vi "Reactor.vi"() -> ()   [LabVIEW 2017]
uses:
  <vilib>/Platform/TimedLoop/XDataNode/timing_clust.ctl
  <vilib>/Platform/TimedLoop/XDataNode/nitl_modes.ctl
  <vilib>/Platform/TimedLoop/XDataNode/wakeup.ctl
  <vilib>/Analysis/baseanly.llb/Mean (DBL).vi
  <vilib>/Utility/file.llb/Read Delimited Spreadsheet (DBL).vi
  <vilib>/platform/TimedLoop/XDataNode/XDataNode.xnode
  <vilib>/Analysis/NI_AALBase.lvlib
  <vilib>/Platform/TimedLoop/XDataNode/XDNodeRunTimeDep.lvlib
panel:
  in  "stop":bool
  in  "Controller":string(combo)
  in  "Controller\nReset":bool
  out "Server Connection":bool
  in  "Stop Reading":bool
  out "System Time [s]":sgl
  out "Power Output":dbl(graph)
  out "Frequency [Hz]":sgl(slide) scale=0.0..60.0
  out "Frequency [Hz]":sgl(slide) scale=0.0..60.0
  out "Frequency [Hz]":sgl(knob) scale=0.0..45.0
  out "Power [W]":dbl(slide) caption="Power Output [W]" scale=0.0..10000.0
  in  "Desired Power [W]":dbl format="%.1f"
  out "WT-10":sgl format="%.1f"
  out "BT-11":sgl format="%.1f"
  out "BT-12":sgl format="%.1f"
  out "WT-13":sgl format="%.1f"
  out "CX-10":dbl format="%.1f"
  out "CX-11":dbl format="%.1f"
  out "WT-20":sgl format="%.1f"
  out "BT-21":sgl format="%.1f"
  out "WT-22":sgl format="%.1f"
  out "BT-23":sgl format="%.1f"
  out "WT-24":sgl format="%.1f"
  out "BT-25":sgl format="%.1f"
  out "WT-26":sgl format="%.1f"
  out "BT-27":sgl format="%.1f"
  out "WT-28":sgl format="%.1f"
  out "BT-29":sgl format="%.1f"
  out "BT-30":sgl format="%.1f"
  out "WT-31":sgl format="%.1f"
  out "BT-32":sgl format="%.1f"
  out "WT-33":sgl format="%.1f"
  out "BT-34":sgl format="%.1f"
  out "WT-35":sgl format="%.1f"
  out "WT-40":sgl format="%.1f"
  out "BT-41":sgl format="%.1f"
  out "WT-42":sgl format="%.1f"
  out "BT-43":sgl format="%.1f"
  out "BT-60":sgl format="%.1f"
  out "WT-61":sgl format="%.1f"
  out "WT-62":sgl format="%.1f"
  out "BT-63":sgl format="%.1f"
  out "WT-64":sgl format="%.1f"
  out "BT-65":sgl format="%.1f"
  out "BT-66":sgl format="%.1f"
  out "WT-67":sgl format="%.1f"
  out "ST-10":sgl format="%.1f"
  out "ST-11":sgl format="%.1f"
  out "ST-12":sgl[](array[numeric]) format="%.1f"
  out "ST-13":sgl format="%.1f"
  out "ST-14":sgl[](array[numeric]) format="%.1f"
  out "AT-01":sgl format="%.1f"
  out "AT-02":sgl format="%.1f"
  in  "Power Output On":bool
  in  "ACTIVATE - CTAH":bool
  in  "CTAH Frequency [Hz]":sgl format="%.1f"
  in  "ACTIVATE - TCHX":bool
  in  "TCHX Frequency [Hz]":sgl format="%.1f"
  in  "ACTIVATE - PUMP":bool
  in  "Pump Frequency [Hz]":sgl format="%.1f"
  out "DHX Primary Flow\n\n\nFM-20 [kg/s]":sgl format="%.3f"
  out "Bypass Flow\n\n\nFM-30 [kg/s]":sgl format="%.3f"
  out "Primary Flow\n\n\nFM-40 [kg/s]":sgl format="%.3f"
  out "DRACS Flow\n\n\nFM-60 [kg/s]":sgl format="%.3f"
  in  "Flow Data?":bool=TRUE
  out "System Safe":bool
  in  "Exit Profile":bool
  in  "Select Operation Mode":T1(ring) caption="Select Operation Mode2"
  out "System Loop Time (ms)":u32
  in  "Load Power Profile":bool
  in  "Dyn. Power Profile File":path
  out "CTAH Temperatures":cluster{"CTAH Outlet":dbl, "CTAH Inlet":dbl}(graph)
  out "CTAH Outlet":dbl format="%0.2f"
  out "CTAH Inlet":dbl format="%0.2f"
  out "Core Temperatures":cluster{"Heater Inlet":dbl, "Heater Outlet":dbl}(graph)
  out "Heater Outlet":dbl format="%0.2f"
  out "Heater Inlet":dbl format="%0.2f"
  out "Profile Step":i32
  out "Power Input Signal [W]":dbl
  out "Output Current 2 [A]":dbl
  out "Output Voltage 2 [V]":dbl
  out "Output Current 1 [A]":dbl
  out "Output Voltage 1 [V]":dbl
  out "Loop Period [ms]":i64
  in  "Pump Operation Mode":i32(listbox)
  in  "TCHX Operation Mode":i32(listbox)
  in  "CTAH Operation Mode":i32(listbox)
  in  "Stop Reactor Interface":bool
  # "DRACS"
  # "PRIMARY"
  # "HOT DRACS"
  # "TCHX"
  # "HOT LEG"
  # "DHX TOP"
  # "N"
  # "COLD DRACS"
  # "DHX"
  # "E"
  # "S"
  # "W"
  # "BYPASS"
  # "N"
  # "CTAH"
  # "SE"
  # "SW"
  # "CTAH Controller"
  # "HEATER"
  # "DHX BOTTOM"
  # "COLD LEG"
  # "PUMP"
  # "Frequency Response Testing"
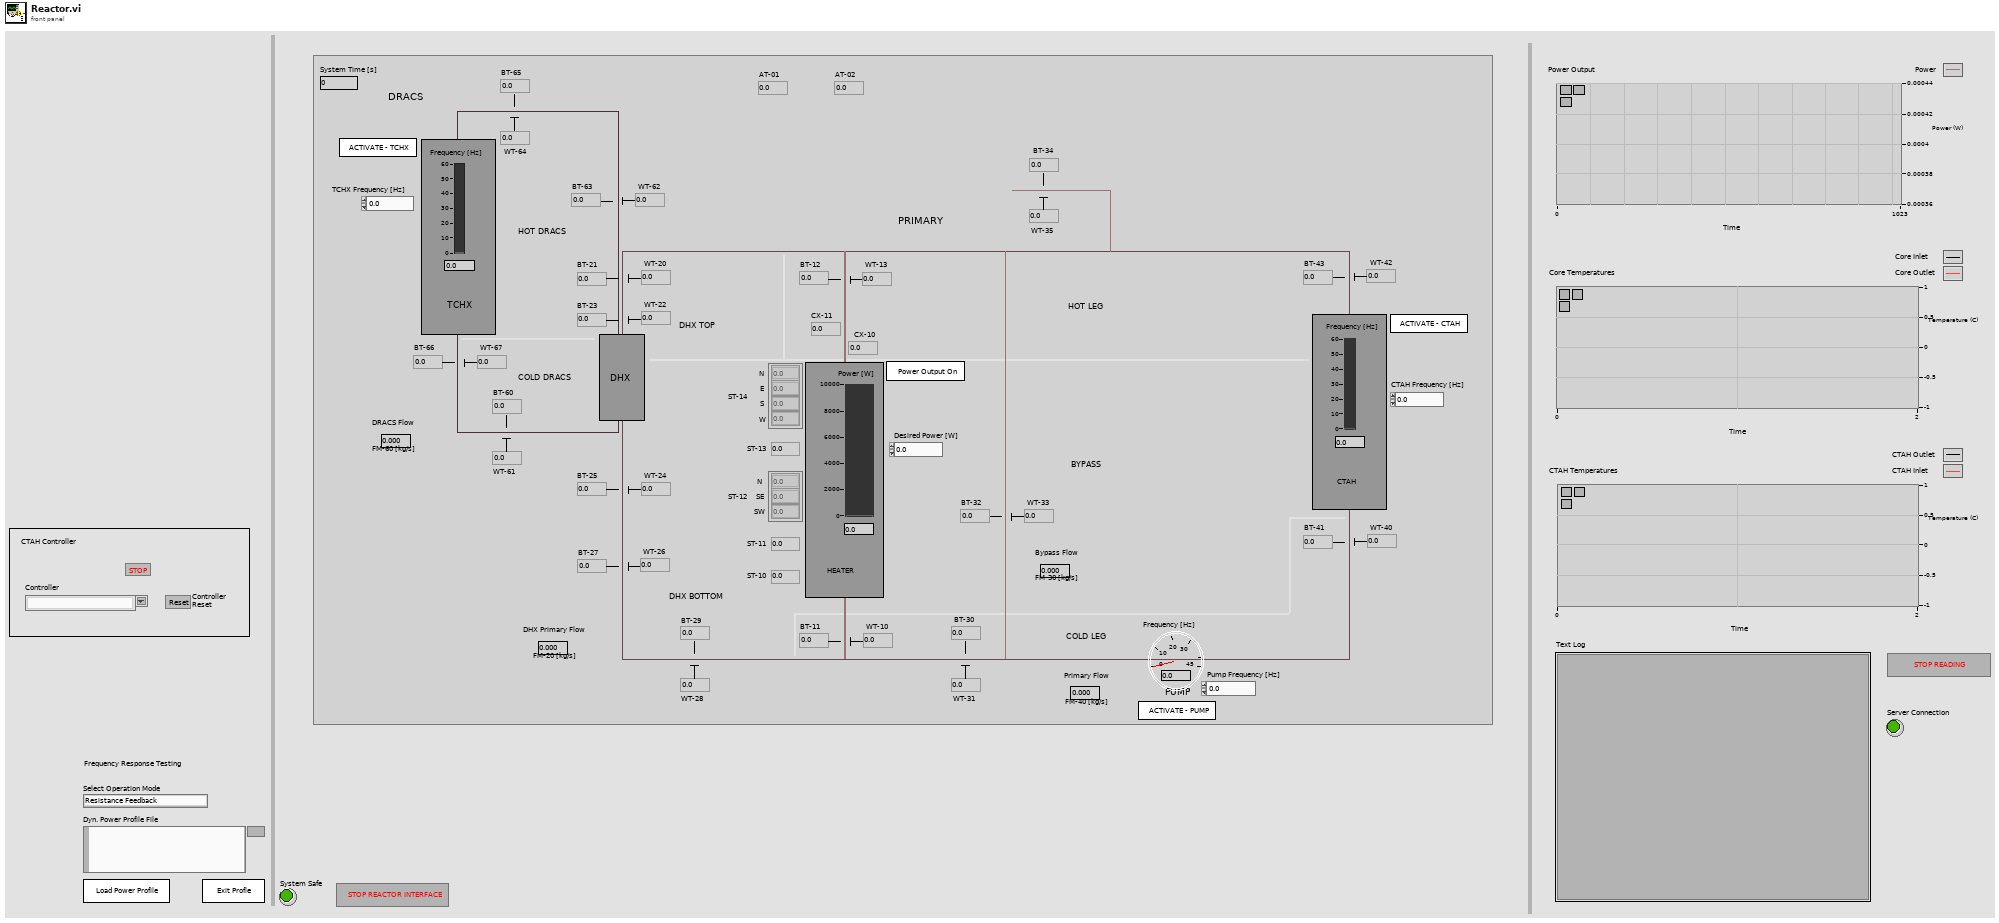
[diagram p1: front panel]
types:
  T1 = enum16{"Resistance Feedback", "Power Profile Input", "Resistance Feedback_Analog", "Power Profile Input_Analog", "Shutdown"}
  T2 = typedef "XDNodeRunTimeDep.lvlib/timing_clust.ctl" = cluster{"Expected End [f-1]":u64, "Actual End [f-1]":u64, "Finished Late? [f-1]":bool, "Expected End [i-1]":u64, "Actual End [i-1]":u64, "Finished Late? [i-1]":bool, "Expected Start [i]":u64, "Actual Start [i]":u64, "Expected Start [f]":u64, "Actual Start [f]":u64, "Source Name":string, "Structure Name":string, "Period":i64, "Deadline":i64, "Offset":i64, "Start":i64, "Priority":i32, "Timeout":i32, "Mode":T3, "Wakeup Reason":T4, "Error":errorcluster, "Source Type":string, "Secondary Source Type":string, "Global End Time":u64, "Global Start Time":u64, "Frame Duration":u64, "Iteration Duration":u64, "Assigned CPU":i32, "I/O Scan Engine Mode":u32}
  T3 = typedef "XDNodeRunTimeDep.lvlib/nitl_modes.ctl" = enum32{"No Change", "Process missed periods, maintain original phase", "Discard missed periods, maintain original phase", "Process missed periods, ignore original phase", "Discard missed periods, ignore original phase"}
  T4 = typedef "XDNodeRunTimeDep.lvlib/wakeup.ctl" = enum32{"Normal", "Aborted", "Asynchronous wakeup", "Timing source error", "Timed loop error", "Timeout"}
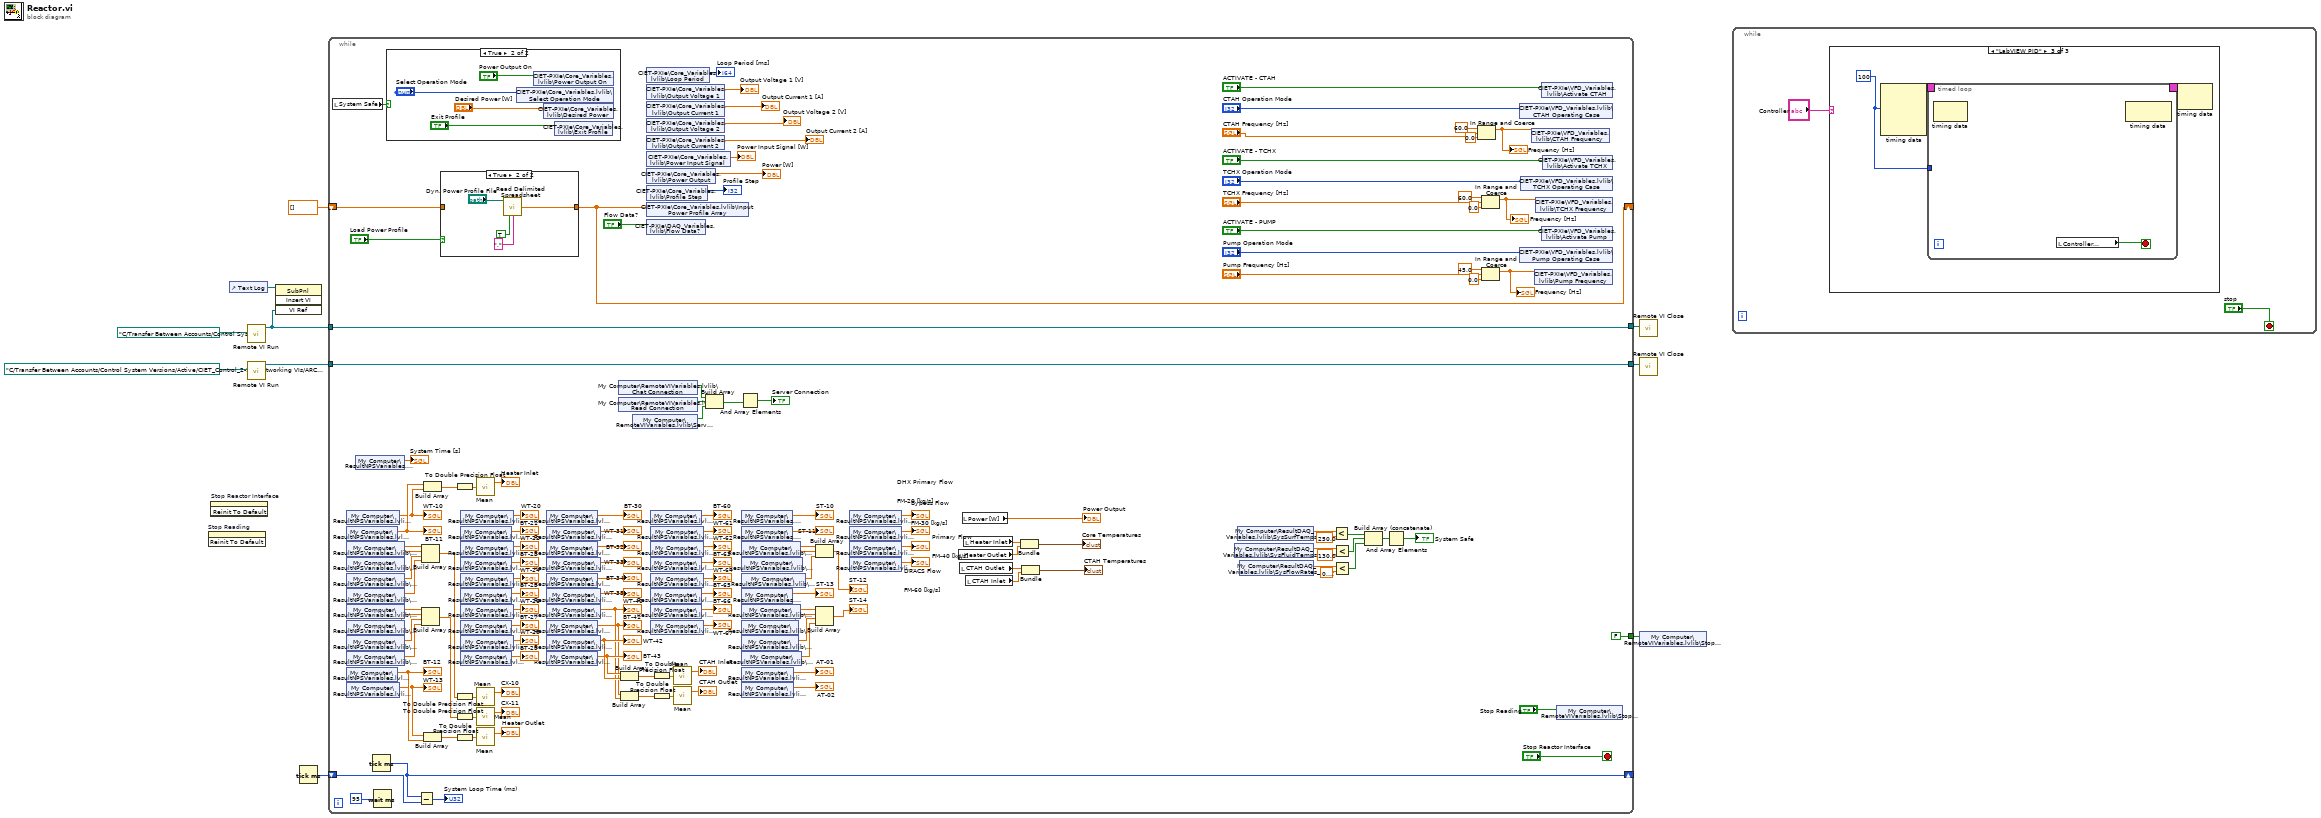
[diagram p0: block diagram]
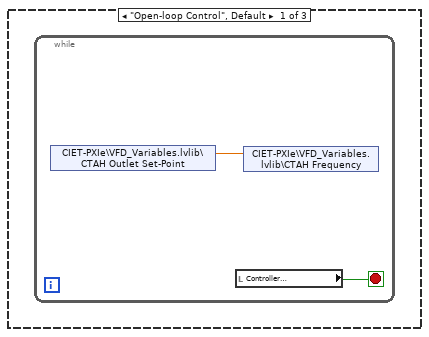
[diagram p2: hidden frame]
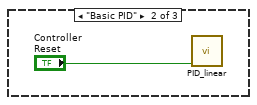
[diagram p3: hidden frame]
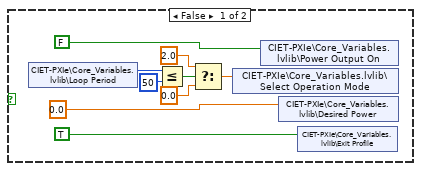
[diagram p4: hidden frame]
diagram:
  n1 = invoke on="Stop Reading" class="Bool (strict)" method="Reinit To Default"() -> ()  [unwired: 3 in, 3 out]
  n2 = invoke on="Stop Reactor Interface" class="Bool (strict)" method="Reinit To Default"() -> ()  [unwired: 3 in, 3 out]
  n3 = control-ref of="Text Log"() -> (w4:refnum<vi>)
  n4 = call "Remote VI Run.vi"("VI Path"=path "C:/Transfer Between Accounts/Control System Versions/Active/CIET_Control_2-1-0/Networking VIs/Updated Chat_Supervisor.vi" ("vi path")) -> ("VI Reference"=w8:refnum<vi>)  [unwired: 10 in]
  n5 = call "Remote VI Run.vi"("VI Path"=path "C:/Transfer Between Accounts/Control System Versions/Active/CIET_Control_2-1-0/Networking VIs/ARCO Reactor Read Client.vi" ("vi path")) -> ("VI Reference"=w6:refnum<vi>)  [unwired: 10 in]
  n6 = invoke on="Invoke Node" class="SubPnl" method="Insert VI"(reference=w4, "VI Ref"=w8) -> ()  [unwired: 2 in, 4 out]
  n7 = Tick Count (ms)() -> (millisecond timer value=w9:u32)
  n8 = while {
    shift-right: [w50] -> _
    shift-left: dbl[] [] ("Input Power Profile Array") -> [w51]
    shift-right: [w48] -> _
    shift-left: w9 -> [w49]
    tunnel: w8 -> [w29]
    tunnel: [w29] -> w7
    tunnel: w6 -> [w27]
    tunnel: [w27] -> w5
    tunnel: [FALSE] -> w1
    stop <- "Stop Reactor Interface" stop-if-true
    n9 = local read "System Safe"() -> (w34:bool)
    n10 = shared-variable "My Computer\\ResultNPSVariables.lvlib\\WT-10_R"() -> (w71:sgl)  [unwired: 1 in, 1 out]
    "WT-10" <- w71
    n11 = shared-variable "My Computer\\ResultNPSVariables.lvlib\\BT-11_R"() -> (w72:sgl)  [unwired: 1 in, 1 out]
    "BT-11" <- w72
    n12 = shared-variable "My Computer\\ResultNPSVariables.lvlib\\CX-10-1_R"() -> (w134:sgl)  [unwired: 1 in, 1 out]
    n13 = shared-variable "My Computer\\ResultNPSVariables.lvlib\\CX-10-2_R"() -> (w133:sgl)  [unwired: 1 in, 1 out]
    n14 = shared-variable "My Computer\\ResultNPSVariables.lvlib\\CX-10-3_R"() -> (w132:sgl)  [unwired: 1 in, 1 out]
    n15 = shared-variable "My Computer\\ResultNPSVariables.lvlib\\CX-10-4_R"() -> (w131:sgl)  [unwired: 1 in, 1 out]
    n16 = shared-variable "My Computer\\ResultNPSVariables.lvlib\\CX-11-1_R"() -> (w127:sgl)  [unwired: 1 in, 1 out]
    n17 = shared-variable "My Computer\\ResultNPSVariables.lvlib\\CX-11-2_R"() -> (w126:sgl)  [unwired: 1 in, 1 out]
    n18 = shared-variable "My Computer\\ResultNPSVariables.lvlib\\CX-11-3_R"() -> (w125:sgl)  [unwired: 1 in, 1 out]
    n19 = shared-variable "My Computer\\ResultNPSVariables.lvlib\\CX-11-4_R"() -> (w124:sgl)  [unwired: 1 in, 1 out]
    n20 = shared-variable "My Computer\\ResultNPSVariables.lvlib\\BT-12_R"() -> (w76:sgl)  [unwired: 1 in, 1 out]
    "BT-12" <- w76
    n21 = shared-variable "My Computer\\ResultNPSVariables.lvlib\\WT-13_R"() -> (w75:sgl)  [unwired: 1 in, 1 out]
    "WT-13" <- w75
    n22 = shared-variable "My Computer\\ResultNPSVariables.lvlib\\Time_R"() -> (→"System Time [s]":sgl)  [unwired: 1 in, 1 out]
    n23 = Tick Count (ms)() -> (millisecond timer value=w48:u32)
    n24 = Wait (ms)(milliseconds to wait=u32 95) -> ()  [unwired: 1 out]
    n25 = case shown="True" w34 {
      frame False {
        n26 = shared-variable "CIET-PXIe\\Core_Variables.lvlib\\Loop Period"() -> (w155:i64)  [unwired: 1 in, 1 out]
        n27 = Less Or Equal?(x=w155, y=i64 50) -> (x <= y?=w156:bool)
        n28 = Select(t=2.0, s=w156, f=0.0) -> (s? t:f=w151:dbl)
        n29 = shared-variable "CIET-PXIe\\Core_Variables.lvlib\\Select Operation Mode"(w151) -> ()  [unwired: 1 in, 1 out]
        n30 = shared-variable "CIET-PXIe\\Core_Variables.lvlib\\Power Output On"(FALSE ("Power Output On")) -> ()  [unwired: 1 in, 1 out]
        n31 = shared-variable "CIET-PXIe\\Core_Variables.lvlib\\Desired Power"(0.0 ("Desired Power")) -> ()  [unwired: 1 in, 1 out]
        n32 = shared-variable "CIET-PXIe\\Core_Variables.lvlib\\Exit Profile"(TRUE ("Exit Profile")) -> ()  [unwired: 1 in, 1 out]
      }
      frame True {
        n33 = shared-variable "CIET-PXIe\\Core_Variables.lvlib\\Select Operation Mode"("Select Operation Mode") -> ()  [unwired: 1 in, 1 out]
        n34 = shared-variable "CIET-PXIe\\Core_Variables.lvlib\\Power Output On"("Power Output On") -> ()  [unwired: 1 in, 1 out]
        n35 = shared-variable "CIET-PXIe\\Core_Variables.lvlib\\Desired Power"("Desired Power [W]") -> ()  [unwired: 1 in, 1 out]
        n36 = shared-variable "CIET-PXIe\\Core_Variables.lvlib\\Exit Profile"("Exit Profile") -> ()  [unwired: 1 in, 1 out]
      }
    }
    n37 = Subtract(x=w48, y=w49) -> (x-y=→"System Loop Time (ms)":u32)
    n38 = Build Array(w134, w133, w132, w131) -> (w130:sgl[])
    n39 = Build Array(w127, w126, w125, w124) -> (w123:sgl[])
    n40 = Build Array(w72, w71) -> (w73:sgl[])
    n41 = Build Array(w75, w76) -> (w77:sgl[])
    n42 = case shown="True" "Load Power Profile" {
      tunnel: [w164 w165] -> w50
      tunnel: w51 -> [w164 _]
      frame False {
      }
      frame True {
        n43 = call-poly <vilib>:"Read Delimited Spreadsheet.vi"("file path (dialog if empty)"="Dyn. Power Profile File", "transpose? (F)"=TRUE, "delimiter (\\t)"="," ("delimiter (\\t)")) -> ("first row"=w165:dbl[])  [unwired: 7 in, 5 out]
      }
    }
    n44 = To Double Precision Float(number=w73) -> (double precision float=w74:dbl[])
    n45 = To Double Precision Float(number=w130) -> (double precision float=w129:dbl[])
    n46 = To Double Precision Float(number=w123) -> (double precision float=w128:dbl[])
    n47 = To Double Precision Float(number=w77) -> (double precision float=w78:dbl[])
    n48 = shared-variable "My Computer\\ResultNPSVariables.lvlib\\WT-20_R"() -> (→"WT-20":sgl)  [unwired: 1 in, 1 out]
    n49 = shared-variable "My Computer\\ResultNPSVariables.lvlib\\BT-21_R"() -> (→"BT-21":sgl)  [unwired: 1 in, 1 out]
    n50 = shared-variable "My Computer\\ResultNPSVariables.lvlib\\WT-22_R"() -> (→"WT-22":sgl)  [unwired: 1 in, 1 out]
    n51 = shared-variable "My Computer\\ResultNPSVariables.lvlib\\BT-23_R"() -> (→"BT-23":sgl)  [unwired: 1 in, 1 out]
    n52 = shared-variable "My Computer\\ResultNPSVariables.lvlib\\WT-24_R"() -> (→"WT-24":sgl)  [unwired: 1 in, 1 out]
    n53 = shared-variable "My Computer\\ResultNPSVariables.lvlib\\BT-25_R"() -> (→"BT-25":sgl)  [unwired: 1 in, 1 out]
    n54 = shared-variable "My Computer\\ResultNPSVariables.lvlib\\WT-26_R"() -> (→"WT-26":sgl)  [unwired: 1 in, 1 out]
    n55 = shared-variable "My Computer\\ResultNPSVariables.lvlib\\BT-27_R"() -> (→"BT-27":sgl)  [unwired: 1 in, 1 out]
    n56 = shared-variable "My Computer\\ResultNPSVariables.lvlib\\WT-28_R"() -> (→"WT-28":sgl)  [unwired: 1 in, 1 out]
    n57 = shared-variable "My Computer\\ResultNPSVariables.lvlib\\BT-29_R"() -> (→"BT-29":sgl)  [unwired: 1 in, 1 out]
    n58 = call-poly <vilib>:"Mean.vi"("X"=w74) -> ("mean"=→"Heater Inlet":dbl)  [unwired: 1 out]
    n59 = call-poly <vilib>:"Mean.vi"("X"=w129) -> ("mean"=→"CX-10":dbl)  [unwired: 1 out]
    n60 = call-poly <vilib>:"Mean.vi"("X"=w128) -> ("mean"=→"CX-11":dbl)  [unwired: 1 out]
    n61 = call-poly <vilib>:"Mean.vi"("X"=w78) -> ("mean"=→"Heater Outlet":dbl)  [unwired: 1 out]
    n62 = shared-variable "My Computer\\ResultNPSVariables.lvlib\\BT-30_R"() -> (→"BT-30":sgl)  [unwired: 1 in, 1 out]
    n63 = shared-variable "My Computer\\ResultNPSVariables.lvlib\\WT-31_R"() -> (→"WT-31":sgl)  [unwired: 1 in, 1 out]
    n64 = shared-variable "My Computer\\ResultNPSVariables.lvlib\\BT-32_R"() -> (→"BT-32":sgl)  [unwired: 1 in, 1 out]
    n65 = shared-variable "My Computer\\ResultNPSVariables.lvlib\\WT-33_R"() -> (→"WT-33":sgl)  [unwired: 1 in, 1 out]
    n66 = shared-variable "My Computer\\ResultNPSVariables.lvlib\\BT-34_R"() -> (→"BT-34":sgl)  [unwired: 1 in, 1 out]
    n67 = shared-variable "My Computer\\ResultNPSVariables.lvlib\\WT-35_R"() -> (→"WT-35":sgl)  [unwired: 1 in, 1 out]
    n68 = shared-variable "My Computer\\ResultNPSVariables.lvlib\\WT-40_R"() -> (w57:sgl)  [unwired: 1 in, 1 out]
    "WT-40" <- w57
    n69 = shared-variable "My Computer\\ResultNPSVariables.lvlib\\BT-41_R"() -> (w56:sgl)  [unwired: 1 in, 1 out]
    "BT-41" <- w56
    n70 = shared-variable "My Computer\\ResultNPSVariables.lvlib\\WT-42_R"() -> (w59:sgl)  [unwired: 1 in, 1 out]
    "WT-42" <- w59
    n71 = shared-variable "My Computer\\ResultNPSVariables.lvlib\\BT-43_R"() -> (w58:sgl)  [unwired: 1 in, 1 out]
    "BT-43" <- w58
    n72 = shared-variable "My Computer\\RemoteVIVariables.lvlib\\Chat Connection"() -> (w26:bool)  [unwired: 1 in, 1 out]
    n73 = shared-variable "My Computer\\RemoteVIVariables.lvlib\\Read Connection"() -> (w25:bool)  [unwired: 1 in, 1 out]
    n74 = Build Array(w58, w59) -> (w64:sgl[])
    n75 = Build Array(w56, w57) -> (w61:sgl[])
    n76 = shared-variable "My Computer\\RemoteVIVariables.lvlib\\Server Status"() -> (w24:bool)  [unwired: 1 in, 1 out]
    n77 = shared-variable "CIET-PXIe\\Core_Variables.lvlib\\Input Power Profile Array"(w50) -> ()  [unwired: 1 in, 1 out]
    n78 = shared-variable "CIET-PXIe\\DAQ_Variables.lvlib\\Flow Data?"("Flow Data?") -> ()  [unwired: 1 in, 1 out]
    n79 = shared-variable "CIET-PXIe\\Core_Variables.lvlib\\Loop Period"() -> (→"Loop Period [ms]":i64)  [unwired: 1 in, 1 out]
    n80 = shared-variable "CIET-PXIe\\Core_Variables.lvlib\\Output Voltage 1"() -> (→"Output Voltage 1 [V]":dbl)  [unwired: 1 in, 1 out]
    n81 = shared-variable "CIET-PXIe\\Core_Variables.lvlib\\Output Current 1"() -> (→"Output Current 1 [A]":dbl)  [unwired: 1 in, 1 out]
    n82 = shared-variable "CIET-PXIe\\Core_Variables.lvlib\\Output Voltage 2"() -> (→"Output Voltage 2 [V]":dbl)  [unwired: 1 in, 1 out]
    n83 = shared-variable "CIET-PXIe\\Core_Variables.lvlib\\Output Current 2"() -> (→"Output Current 2 [A]":dbl)  [unwired: 1 in, 1 out]
    n84 = shared-variable "CIET-PXIe\\Core_Variables.lvlib\\Power Input Signal"() -> (→"Power Input Signal [W]":dbl)  [unwired: 1 in, 1 out]
    n85 = shared-variable "CIET-PXIe\\Core_Variables.lvlib\\Power Output"() -> (→"Power [W]":dbl)  [unwired: 1 in, 1 out]
    n86 = shared-variable "CIET-PXIe\\Core_Variables.lvlib\\Profile Step"() -> (→"Profile Step":i32)  [unwired: 1 in, 1 out]
    n87 = shared-variable "My Computer\\ResultNPSVariables.lvlib\\BT-60_R"() -> (→"BT-60":sgl)  [unwired: 1 in, 1 out]
    n88 = shared-variable "My Computer\\ResultNPSVariables.lvlib\\WT-61_R"() -> (→"WT-61":sgl)  [unwired: 1 in, 1 out]
    n89 = shared-variable "My Computer\\ResultNPSVariables.lvlib\\WT-62_R"() -> (→"WT-62":sgl)  [unwired: 1 in, 1 out]
    n90 = shared-variable "My Computer\\ResultNPSVariables.lvlib\\BT-63_R"() -> (→"BT-63":sgl)  [unwired: 1 in, 1 out]
    n91 = shared-variable "My Computer\\ResultNPSVariables.lvlib\\WT-64_R"() -> (→"WT-64":sgl)  [unwired: 1 in, 1 out]
    n92 = shared-variable "My Computer\\ResultNPSVariables.lvlib\\BT-65_R"() -> (→"BT-65":sgl)  [unwired: 1 in, 1 out]
    n93 = shared-variable "My Computer\\ResultNPSVariables.lvlib\\BT-66_R"() -> (→"BT-66":sgl)  [unwired: 1 in, 1 out]
    n94 = shared-variable "My Computer\\ResultNPSVariables.lvlib\\WT-67_R"() -> (→"WT-67":sgl)  [unwired: 1 in, 1 out]
    n95 = To Double Precision Float(number=w64) -> (double precision float=w65:dbl[])
    n96 = To Double Precision Float(number=w61) -> (double precision float=w62:dbl[])
    n97 = call-poly <vilib>:"Mean.vi"("X"=w65) -> ("mean"=→"CTAH Inlet":dbl)  [unwired: 1 out]
    n98 = call-poly <vilib>:"Mean.vi"("X"=w62) -> ("mean"=→"CTAH Outlet":dbl)  [unwired: 1 out]
    n99 = Build Array(w26, w25, w24) -> (w23:bool[])
    n100 = And Array Elements(Boolean array=w23) -> (logical AND=→"Server Connection":bool)
    n101 = shared-variable "My Computer\\ResultNPSVariables.lvlib\\ST-10_R"() -> (→"ST-10":sgl)  [unwired: 1 in, 1 out]
    n102 = shared-variable "My Computer\\ResultNPSVariables.lvlib\\ST-11_R"() -> (→"ST-11":sgl)  [unwired: 1 in, 1 out]
    n103 = shared-variable "My Computer\\ResultNPSVariables.lvlib\\ST-12-N_R"() -> (w94:sgl)  [unwired: 1 in, 1 out]
    n104 = shared-variable "My Computer\\ResultNPSVariables.lvlib\\ST-12-SE_R"() -> (w93:sgl)  [unwired: 1 in, 1 out]
    n105 = shared-variable "My Computer\\ResultNPSVariables.lvlib\\ST-12-SW_R"() -> (w92:sgl)  [unwired: 1 in, 1 out]
    n106 = shared-variable "My Computer\\ResultNPSVariables.lvlib\\ST-13_R"() -> (→"ST-13":sgl)  [unwired: 1 in, 1 out]
    n107 = shared-variable "My Computer\\ResultNPSVariables.lvlib\\ST-14-N_R"() -> (w89:sgl)  [unwired: 1 in, 1 out]
    n108 = shared-variable "My Computer\\ResultNPSVariables.lvlib\\ST-14-E_R"() -> (w88:sgl)  [unwired: 1 in, 1 out]
    n109 = shared-variable "My Computer\\ResultNPSVariables.lvlib\\ST-14-S_R"() -> (w87:sgl)  [unwired: 1 in, 1 out]
    n110 = shared-variable "My Computer\\ResultNPSVariables.lvlib\\ST-14-W_R"() -> (w86:sgl)  [unwired: 1 in, 1 out]
    n111 = shared-variable "My Computer\\ResultNPSVariables.lvlib\\AT-01_R"() -> (→"AT-01":sgl)  [unwired: 1 in, 1 out]
    n112 = shared-variable "My Computer\\ResultNPSVariables.lvlib\\AT-02_R"() -> (→"AT-02":sgl)  [unwired: 1 in, 1 out]
    n113 = Build Array(w94, w93, w92) -> (→"ST-12":sgl[])
    n114 = Build Array(w89, w88, w87, w86) -> (→"ST-14":sgl[])
    n115 = shared-variable "My Computer\\ResultNPSVariables.lvlib\\FM-20_R"() -> (→"DHX Primary Flow\n\n\nFM-20 [kg/s]":sgl)  [unwired: 1 in, 1 out]
    n116 = shared-variable "My Computer\\ResultNPSVariables.lvlib\\FM-30_R"() -> (→"Bypass Flow\n\n\nFM-30 [kg/s]":sgl)  [unwired: 1 in, 1 out]
    n117 = shared-variable "My Computer\\ResultNPSVariables.lvlib\\FM-40_R"() -> (→"Primary Flow\n\n\nFM-40 [kg/s]":sgl)  [unwired: 1 in, 1 out]
    n118 = shared-variable "My Computer\\ResultNPSVariables.lvlib\\FM-60_R"() -> (→"DRACS Flow\n\n\nFM-60 [kg/s]":sgl)  [unwired: 1 in, 1 out]
    n119 = local read "Heater Outlet"() -> (w66:dbl)
    n120 = local read "CTAH Outlet"() -> (w54:dbl)
    n121 = local read "Power [W]"() -> (→"Power Output":dbl)
    n122 = local read "Heater Inlet"() -> (w67:dbl)
    n123 = local read "CTAH Inlet"() -> (w53:dbl)
    n124 = Bundle("Heater Inlet"=w67, "Heater Outlet"=w66) -> (→"Core Temperatures":cluster{"Heater Inlet":dbl, "Heater Outlet":dbl})  [unwired: 1 in]
    n125 = Bundle("CTAH Outlet"=w54, "CTAH Inlet"=w53) -> (→"CTAH Temperatures":cluster{"CTAH Outlet":dbl, "CTAH Inlet":dbl})  [unwired: 1 in]
    n126 = shared-variable "My Computer\\ResultDAQ_Variables.lvlib\\SysFluidTemps_R"() -> (w40:sgl[])  [unwired: 1 in, 1 out]
    n127 = shared-variable "My Computer\\ResultDAQ_Variables.lvlib\\SysSurfTemps_R"() -> (w42:sgl[])  [unwired: 1 in, 1 out]
    n128 = shared-variable "My Computer\\ResultDAQ_Variables.lvlib\\SysFlowRates_R"() -> (w38:sgl[])  [unwired: 1 in, 1 out]
    n129 = Less?(x=w42, y=sgl 250.0) -> (x < y?=w44:bool[])
    n130 = Less?(x=w40, y=sgl 130.0) -> (x < y?=w37:bool[])
    n131 = Less?(x=w38, y=sgl 0.2) -> (x < y?=w36:bool[])
    n132 = Build Array (concatenate)(w44, w37, w36) -> (w45:bool[])
    n133 = And Array Elements(Boolean array=w45) -> (logical AND=→"System Safe":bool)
    n134 = In Range and Coerce(upper limit=sgl 60.0, x="CTAH Frequency [Hz]", lower limit=sgl 0.0) -> (coerced(x)=w15:sgl)  [unwired: 1 out]
    "Frequency [Hz]" <- w15
    n135 = In Range and Coerce(upper limit=sgl 60.0, x="TCHX Frequency [Hz]", lower limit=sgl 0.0) -> (coerced(x)=w14:sgl)  [unwired: 1 out]
    "Frequency [Hz]" <- w14
    n136 = In Range and Coerce(upper limit=sgl 45.0, x="Pump Frequency [Hz]", lower limit=sgl 0.0) -> (coerced(x)=w13:sgl)  [unwired: 1 out]
    "Frequency [Hz]" <- w13
    n137 = shared-variable "CIET-PXIe\\VFD_Variables.lvlib\\CTAH Operating Case"("CTAH Operation Mode") -> ()  [unwired: 1 in, 1 out]
    n138 = shared-variable "CIET-PXIe\\VFD_Variables.lvlib\\Pump Operating Case"("Pump Operation Mode") -> ()  [unwired: 1 in, 1 out]
    n139 = shared-variable "CIET-PXIe\\VFD_Variables.lvlib\\TCHX Operating Case"("TCHX Operation Mode") -> ()  [unwired: 1 in, 1 out]
    n140 = shared-variable "CIET-PXIe\\VFD_Variables.lvlib\\CTAH Frequency"(w15) -> ()  [unwired: 1 in, 1 out]
    n141 = shared-variable "CIET-PXIe\\VFD_Variables.lvlib\\Pump Frequency"(w13) -> ()  [unwired: 1 in, 1 out]
    n142 = shared-variable "CIET-PXIe\\VFD_Variables.lvlib\\TCHX Frequency"(w14) -> ()  [unwired: 1 in, 1 out]
    n143 = shared-variable "CIET-PXIe\\VFD_Variables.lvlib\\Activate CTAH"("ACTIVATE - CTAH") -> ()  [unwired: 1 in, 1 out]
    n144 = shared-variable "CIET-PXIe\\VFD_Variables.lvlib\\Activate Pump"("ACTIVATE - PUMP") -> ()  [unwired: 1 in, 1 out]
    n145 = shared-variable "CIET-PXIe\\VFD_Variables.lvlib\\Activate TCHX"("ACTIVATE - TCHX") -> ()  [unwired: 1 in, 1 out]
    n146 = shared-variable "My Computer\\RemoteVIVariables.lvlib\\Stop Reading"("Stop Reading") -> ()  [unwired: 1 in, 1 out]
  }
  n147 = call "Remote VI Close.vi"("reference"=w7) -> ()  [unwired: 10 in, 1 out]
  n148 = call "Remote VI Close.vi"("reference"=w5) -> ()  [unwired: 10 in, 1 out]
  n149 = shared-variable "My Computer\\RemoteVIVariables.lvlib\\Stop Reading"(w1) -> ()  [unwired: 1 in, 1 out]
  n150 = while {
    stop <- "stop" stop-if-true
    n151 = case shown="\"LabVIEW PID\"" "Controller" {
      frame "Open-loop Control", Default {
        n152 = while {
          stop <- w172 stop-if-true
          n153 = shared-variable "CIET-PXIe\\VFD_Variables.lvlib\\CTAH Outlet Set-Point"() -> (w171:dbl)  [unwired: 1 in, 1 out]
          n154 = local read "Controller\nReset"() -> (w172:bool)
          n155 = shared-variable "CIET-PXIe\\VFD_Variables.lvlib\\CTAH Frequency"(w171) -> ()  [unwired: 1 in, 1 out]
        }
      }
      frame "Basic PID" {
        n156 = call "PID_linear.vi"("Stop Controller Loop"="Controller\nReset") -> ()  [unwired: 11 in]
      }
      frame "LabVIEW PID" {
        w174 = 100
        n157 = node-c288(w174) -> (w176:T2)  [unwired: 3 in]
        n158 = timed-loop {
          timing: w176 -> [_]
          timing-out: [_] -> w175
          tunnel: w174 -> [_]
          stop <- w177 stop-if-true
          n159 = node-c288() -> ()  [unwired: 1 in, 1 out]
          n160 = local read "Controller\nReset"() -> (w177:bool)
          n161 = node-c288() -> ()  [unwired: 1 in, 1 out]
        }
        n162 = node-c288(w175) -> ()  [unwired: 1 out]
      }
    }
  }
